vi "QuickLoadData.vi"(3 "Fileformat":enum16{"Herty", "Ken"}(ring), 5 "Path":refnum<vi>) -> (0 "gap photons":u32, 1 "invalid photons":u32, 2 "total":u32)   [LabVIEW 2009]
panel:
  out "%done":dbl(slide) scale=0.0..100.0
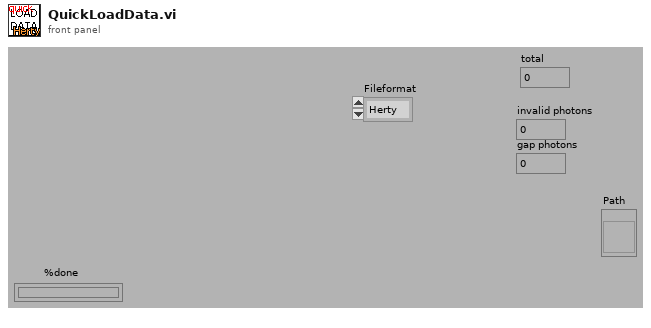
[diagram p1: front panel]
types:
  T1 = typedef "FIFOSettings_BH.ctt" = cluster{"Measurement":cluster{"Binning (ms)":sgl, "External Trigger Condition":u16, "Stop Condition:":u16, "Stop Count":dbl, "Buffer Size (Photons)":u16, "No of Channels":u16, "Ext Latch Delay":i16}, "ADC":cluster{"Module":u16, "ADC Resolution":i32, "Dither Range":i16, "Count Increment":i16, "Macro Time Clock":i16}, "SYNC":cluster{"SYNC ZC Level (mV)":sgl, "SYNC Freq Divider":i16, "SYNC Holdoff (ns)":sgl, "SYNC Threshold (mV)":sgl}, "TAC":cluster{"TAC Range (ns)":sgl, "TAC Gain":i16, "TAC Offset (%)":sgl, "TAC Limit Low (%)":sgl, "TAC Limit High (%)":sgl}, "CFD":cluster{"CFD Limit Low (mV)":sgl, "CFD Limit High (mV)":sgl, "CFD ZC Level (mV)":sgl, "CFD Holdoff (ns)":sgl}}
  T2 = typedef "ImageCluster.ctl" = cluster{"decay":u16[][][][][], "sum of photons":u32[][][][]}
  T3 = cluster{"router channels":u8[], "macro times":dbl[], "micro times":u16[], "invalid times":dbl[], "gap times":dbl[]}
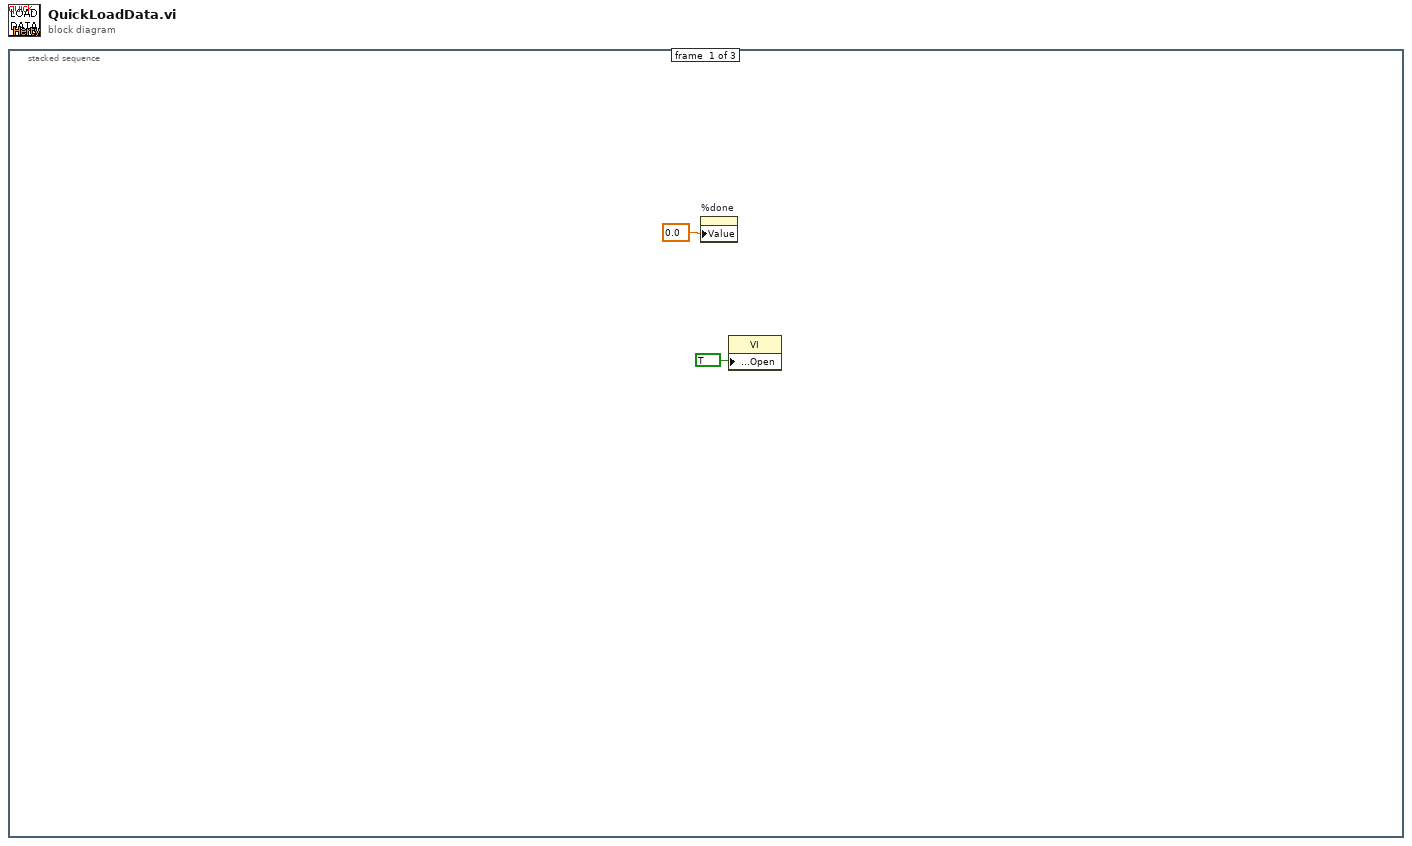
[diagram p0: block diagram]
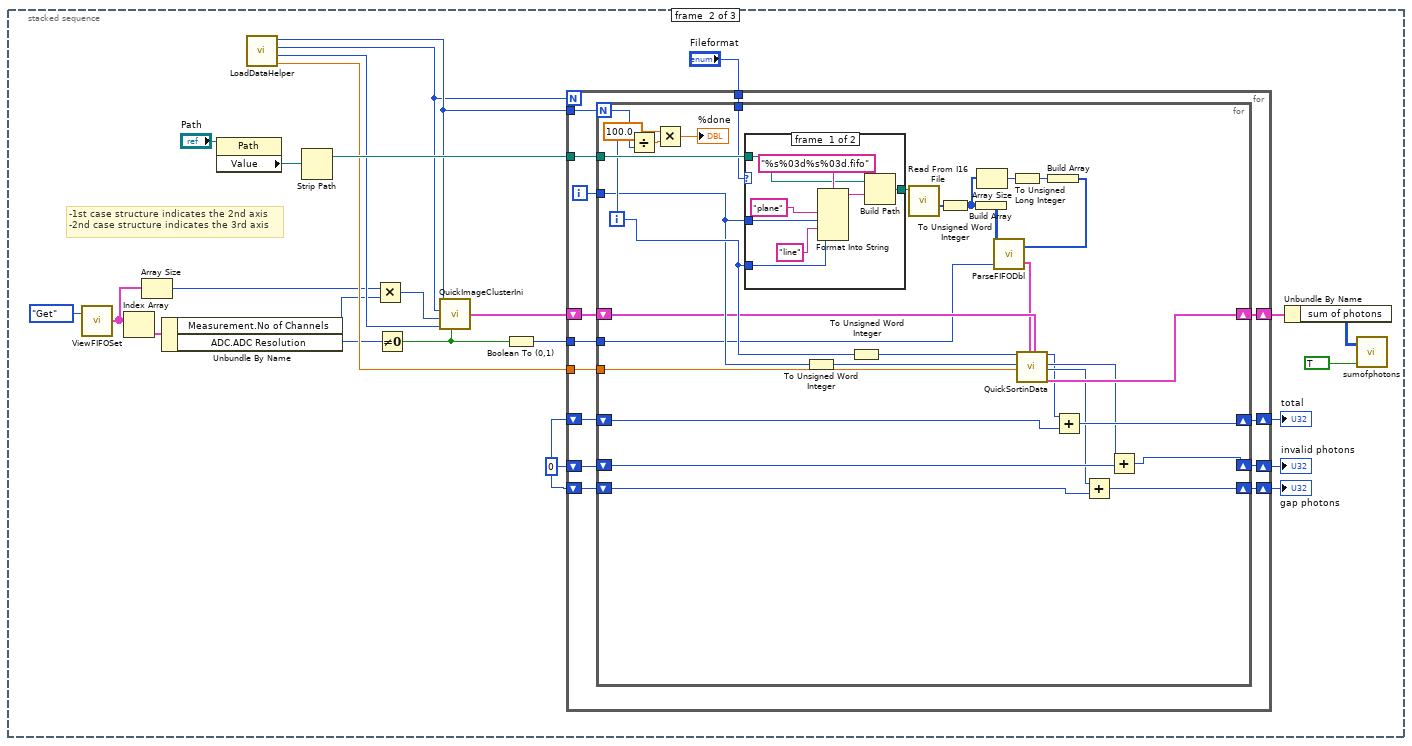
[diagram p2: hidden frame]
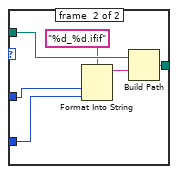
[diagram p3: hidden frame]
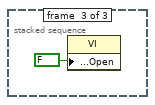
[diagram p4: hidden frame]
diagram:
  n1 = stacked-sequence {
    frame #0 {
      n2 = property on="%done" class="Slide (strict)"("Value"=0.0 ("%done")) -> ()  [unwired: 2 in, 2 out]
      n3 = property class="VI"("Front Panel Window:Open"=TRUE) -> ()  [unwired: 2 in, 2 out]
    }
    frame #1 {
      w20 = u32 0
      # "-1st case structure indicates the 2nd axis\n-2nd case structure indicates the 3rd axis"
      n4 = call "ViewFIFOSet.vi"("Enum"=enum16{"Display", "change", "Get", "Set"}."Get") -> ("FIFO Settings (Array)"=w6:T1[])  [unwired: 1 in]
      n5 = Index Array(array=w6) -> (element=w8:T1)  [unwired: 1 in]
      n6 = Array Size(array=w6) -> (size(s)=w4:i32)
      n7 = Unbundle By Name(w8) -> ("Measurement.No of Channels"=w5:u16, "ADC.ADC Resolution"=w7:i32)
      n8 = property on="Property Node" class="Path"(reference="Path") -> ("Value"=w26:path)  [unwired: 1 in, 2 out]
      n9 = call "LoadDataHelper.vi"() -> ("Time Resolution [ms/pixel]"=w18:dbl, "pixel per line"=w15:u32, "planes"=w14:u32, "lines"=w16:u32)  [unwired: 7 in, 1 out]
      n10 = Strip Path(path=w26) -> (stripped path=w24:path)  [unwired: 1 out]
      n11 = Multiply(x=w4, y=w5) -> (x*y=w3:i32)
      n12 = Not Equal To 0?(x=w7) -> (x != 0?=w17:bool)
      n13 = call "QuickImageClusterIni.vi"("lines"=w16, "planes"=w14, "No. of Channels"=w3, "pixel per line"=w15, "48bit?"=w17) -> ("IMAGE Cluster"=w23:T2)
      n14 = Boolean To (0,1)(Boolean=w17) -> (0, 1=w9:i16)
      n15 = for {
        N: w14 -> [_]
        tunnel: w16 -> [w38]
        tunnel: w24 -> [w41]
        tunnel: w9 -> [w39]
        tunnel: w18 -> [w37]
        shift-right: [w35] -> w12
        shift-left: w23 -> [w36]
        shift-right: [w32] -> w22
        shift-left: w20 -> [w34]
        shift-right: [w31] -> w21
        shift-left: w20 -> [w33]
        shift-right: [w30] -> w19
        shift-left: w20 -> [w29]
        tunnel: "Fileformat" -> [w28]
        i -> [w40]
        n16 = for {
          N: w38 -> [w51]
          tunnel: w41 -> [w72]
          tunnel: w40 -> [w70]
          tunnel: w39 -> [w47]
          tunnel: w37 -> [w69]
          shift-right: [w67] -> w35
          shift-left: w36 -> [w68]
          shift-right: [w66] -> w32
          shift-left: w34 -> [w64]
          shift-right: [w65] -> w31
          shift-left: w33 -> [w63]
          shift-right: [w62] -> w30
          shift-left: w29 -> [w61]
          tunnel: w28 -> [w60]
          i -> [w71]
          n17 = Divide(x=w71, y=w51) -> (x/y=w50:dbl)
          n18 = Multiply(x=100.0, y=w50) -> (x*y=→"%done":dbl)
          n19 = case shown="\"Herty\", Default" w60 {
            tunnel: w72 -> [w77 w86]
            tunnel: [w75 w84] -> w59
            tunnel: w71 -> [w74 w82]
            tunnel: w70 -> [w73 w83]
            frame #0 {
              n20 = Format Into String(format string="%s%03d%s%03d.fifo", "plane", w73, "line", w74) -> (resulting string=w76:string)  [unwired: 2 in, 1 out]
              n21 = Build Path(base path=w77, name or relative path=w76) -> (appended path=w75:path)
            }
            frame #1 {
              n22 = Format Into String(format string="%d_%d.ifif", w83, w82) -> (resulting string=w85:string)  [unwired: 2 in, 1 out]
              n23 = Build Path(base path=w86, name or relative path=w85) -> (appended path=w84:path)
            }
          }
          n24 = To Unsigned Word Integer(number=w70) -> (unsigned 16bit integer=w52:u16)
          n25 = To Unsigned Word Integer(number=w71) -> (unsigned 16bit integer=w53:u16)
          n26 = call "Read From I16 File.vi"("file path (dialog if empty)"=w59) -> ("1D array"=w58:i16[])  [unwired: 6 in, 4 out]
          n27 = To Unsigned Word Integer(number=w58) -> (unsigned 16bit integer=w45:u16[])
          n28 = Build Array(w45) -> (w46:u16[][])
          n29 = Array Size(array=w45) -> (size(s)=w44:i32)
          n30 = To Unsigned Long Integer(number=w44) -> (unsigned 32bit integer=w43:u32)
          n31 = Build Array(w43) -> (w42:u32[])
          n32 = call "ParseFIFODbl.vi"("photoncount"=w42, "SPC Format"=w47, "FIFO rawdata"=w46) -> ("rawdata"=w54:T3)
          n33 = call "QuickSortinData.vi"("line"=w53, "plane"=w52, "binning [ms]"=w69, "rawdata"=w54, "IMAGE Cluster 4"=w68) -> ("valid"=w55:i32, "invalid"=w57:u32, "gap"=w56:u32, "IMAGE Cluster"=w67:T2)  [unwired: 11 in]
          n34 = Add(x=w55, y=w61) -> (x+y=w62:u32)
          n35 = Add(x=w56, y=w63) -> (x+y=w65:u32)
          n36 = Add(x=w57, y=w64) -> (x+y=w66:u32)
        }
      }
      "invalid photons" <- w22
      "gap photons" <- w21
      "total" <- w19
      n37 = Unbundle By Name(w12) -> ("sum of photons"=w10:u32[][][][])
      n38 = call "sumofphotons.vi"("s"=TRUE, "sum of photons"=w10) -> ()  [unwired: 1 out]
    }
    frame #2 {
      n39 = property class="VI"("Front Panel Window:Open"=FALSE) -> ()  [unwired: 2 in, 2 out]
    }
  }
